vi "Strings to Master Configuration.vi"(11 "Gas":string[][](array[string])) -> (3 "Gas Sequence":T1[](array[typedef]))   [LabVIEW 2015]
uses:
  Tests/Controls/Gas Info.ctl
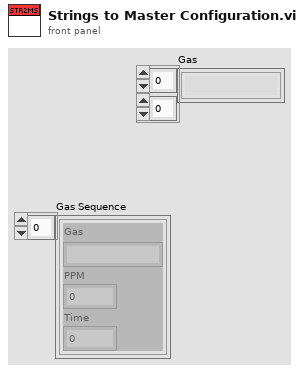
[diagram p1: front panel]
types:
  T1 = typedef "Gas Info.ctl" = cluster{"Gas":string, "PPM":dbl, "Time":u32}
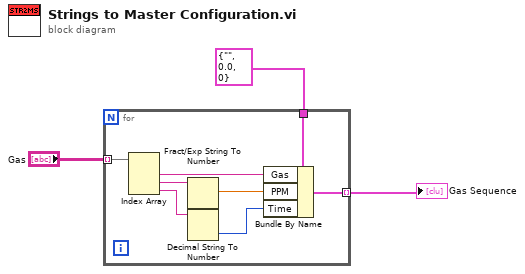
[diagram p0: block diagram]
diagram:
  n1 = for {
    tunnel: "Gas" -> [w11] mode=indexing
    tunnel: T1 {"Gas"="", "PPM"=0.0, "Time"=0} ("Gas Info") -> [w7]
    tunnel: [w6] -> w1 mode=indexing
    n2 = Index Array(array=w11) -> (element #1=w10:string, element #2=w9:string, element #3=w5:string)  [unwired: 3 in]
    n3 = Fract/Exp String To Number(string=w9) -> (number=w8:dbl)  [unwired: 3 in, 1 out]
    n4 = Decimal String To Number(string=w5) -> (number=w4:i32)  [unwired: 2 in, 1 out]
    n5 = Bundle By Name(cluster=w7, "Gas"=w10, "PPM"=w8, "Time"=w4) -> (w6:T1)
  }
  "Gas Sequence" <- w1
